vi "LvMPDC_SUB_ListDirectory.vi"(8 "error in (no error)":errorcluster, 10 "dir path":path, 11 "Connect ID":refnum<k5>) -> (0 "error out":errorcluster, 1 "file path[]":path[](array[path]), 2 "dir path[]":path[](array[path]), 3 "Connect ID out":refnum<k5>)   [LabVIEW 2012]
panel:
  # "LvMPDC:: ListDirectory"
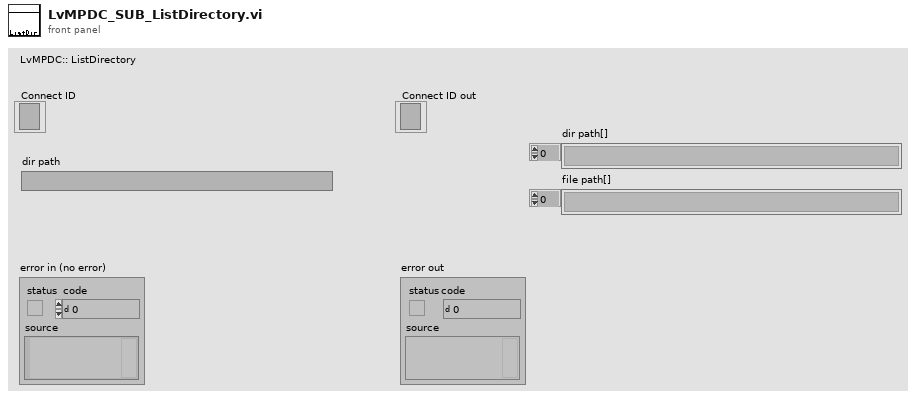
[diagram p1: front panel]
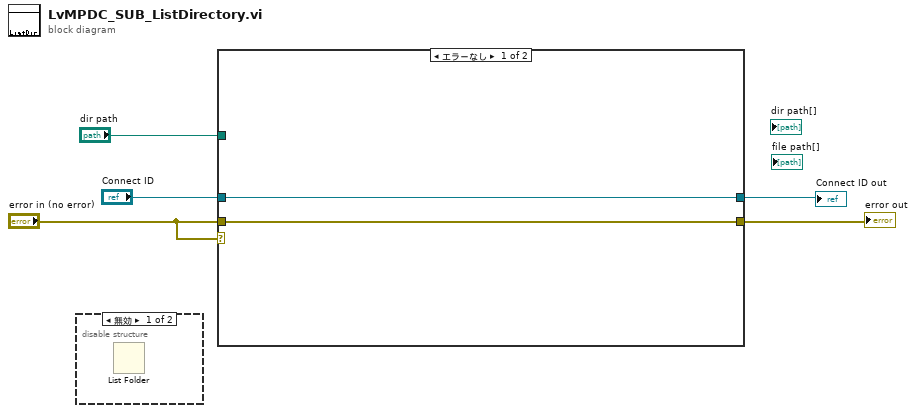
[diagram p0: block diagram]
diagram:
  n1 = disable-structure shown="無効" {
    frame Disabled {
      n2 = List Folder() -> ()  [unwired: 4 in, 4 out]
    }
    frame Enabled {
    }
  }
  n3 = case shown="エラーなし" "error in (no error)" {
    tunnel: "Connect ID" -> [w6 w9]
    tunnel: "error in (no error)" -> [w7 w8]
    tunnel: [w6 w9] -> w4
    tunnel: [w7 w8] -> w3
    tunnel: "dir path" -> [_ _]
    frame No Error {
    }
    frame Error {
    }
  }
  "Connect ID out" <- w4
  "error out" <- w3
